vi "Unit 5M.vi"() -> ()   [LabVIEW 2023]
panel:
  out "isTrue":bool=TRUE
  in  "Мащаб 1 сек:1":u32=1000
  in  "k Минути":dbl format="%#_2g"
  out "Nк %":dbl format="%#_4g"
  out "Минути":dbl format="%#_2g"
  out "Час":i64
  out "tmp":dbl
  out "Часа":dbl format="%#_2g"
  out "Минути":dbl format="%#_4g"
  out "dN %/мин":dbl format="%#_2g"
  in  "dN/dT %/ h":dbl format="%#_2g"
  in  "N1 %":dbl format="%#_3g"
  out "Waveform Chart":T1(graph)
  out "N след 1 минута":dbl format="%#_4g"
  out "N текуща %":dbl format="%#_4g"
  in  "N2 %":dbl format="%#_3g"
  # "със"
  # "За"
  # "min"
  # "мил. сек."
  # "след"
  # "Общо време"
  # ":"
  # "="
  # "%"
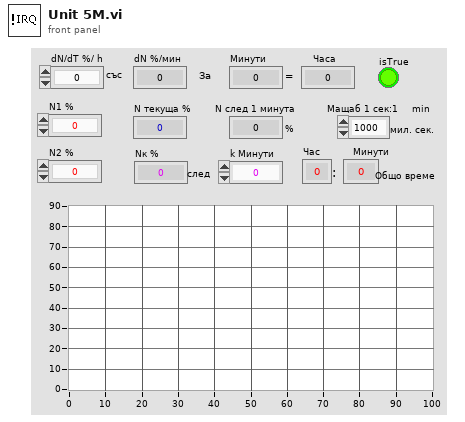
[diagram p1: front panel]
types:
  T1 = cluster{"N текуща % ":dbl, "N2 % ":dbl, "Nк %  ":dbl}
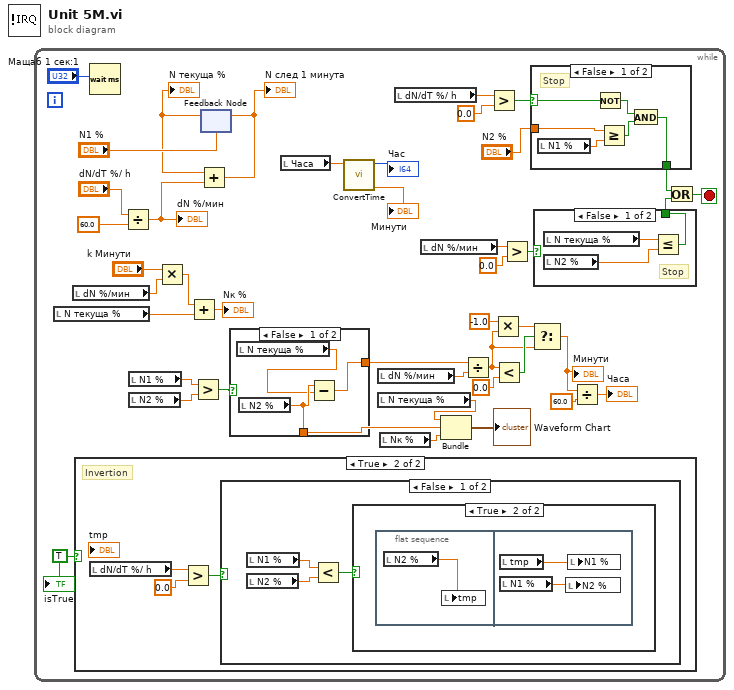
[diagram p0: block diagram]
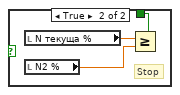
[diagram p2: hidden frame]
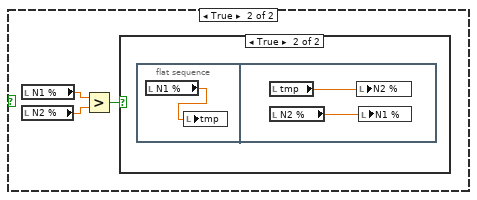
[diagram p5: hidden frame]
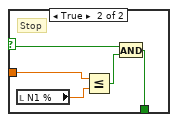
[diagram p7: hidden frame]
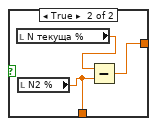
[diagram p8: hidden frame]
diagram:
  n1 = while {
    stop <- w6 stop-if-true
    w27 = TRUE
    n2 = local read "N текуща %"() -> (w9:dbl)
    n3 = local read "dN %/мин"() -> (w12:dbl)
    n4 = case shown="True" w27 {
      frame False {
      }
      frame True {
        # "Invertion"
        n5 = local read "dN/dT %/ h"() -> (w52:dbl)
        n6 = Greater?(x=w52, y=0.0) -> (0:w50:bool)
        n7 = case shown="False" w50 {
          frame False {
            n8 = local read "N1 %"() -> (w55:dbl)
            n9 = local read "N2 %"() -> (w54:dbl)
            n10 = Less?(x=w55, y=w54) -> (x < y?=w53:bool)
            n11 = case shown="True" w53 {
              frame False {
              }
              frame True {
                n12 = flat-sequence {
                  frame #0 {
                    n13 = local read "N2 %"() -> (w56:dbl)
                    n14 = local write "tmp"(w56) -> ()
                  }
                  frame #1 {
                    n15 = local read "tmp"() -> (w57:dbl)
                    n16 = local read "N1 %"() -> (w58:dbl)
                    n17 = local write "N2 %"(w58) -> ()
                    n18 = local write "N1 %"(w57) -> ()
                  }
                }
              }
            }
          }
          frame True {
            n19 = local read "N1 %"() -> (w61:dbl)
            n20 = local read "N2 %"() -> (w60:dbl)
            n21 = Greater?(x=w61, y=w60) -> (0:w59:bool)
            n22 = case shown="True" w59 {
              frame False {
              }
              frame True {
                n23 = flat-sequence {
                  frame #0 {
                    n24 = local read "N1 %"() -> (w62:dbl)
                    n25 = local write "tmp"(w62) -> ()
                  }
                  frame #1 {
                    n26 = local read "tmp"() -> (w64:dbl)
                    n27 = local read "N2 %"() -> (w63:dbl)
                    n28 = local write "N2 %"(w64) -> ()
                    n29 = local write "N1 %"(w63) -> ()
                  }
                }
              }
            }
          }
        }
      }
    }
    n30 = Wait (ms)(milliseconds to wait="Мащаб 1 сек:1") -> ()  [unwired: 1 out]
    n31 = Divide(x="dN/dT %/ h", y=60.0) -> (x/y=w40:dbl)
    "dN %/мин" <- w40
    n32 = local read "N1 %"() -> (w36:dbl)
    n33 = local read "N2 %"() -> (w35:dbl)
    n34 = Multiply(x="k Минути", y=w12) -> (x*y=w10:dbl)
    n35 = Add(x=w10, y=w9) -> (x+y=→"Nк %":dbl)
    n36 = Greater?(x=w36, y=w35) -> (0:w34:bool)
    n37 = feedback #1("N1 %") -> (w39:dbl)
    "N текуща %" <- w39
    n38 = Add(x=w39, y=w40) -> (x+y=w38:dbl)
    "N след 1 минута" <- w38
    n39 = feedback-in #1(w38) -> ()
    n40 = case shown="False" w34 {
      tunnel: [w78 w81] -> w33
      tunnel: [w77 w79] -> w30
      frame False {
        n41 = local read "N текуща %"() -> (w76:dbl)
        n42 = local read "N2 %"() -> (w77:dbl)
        n43 = Subtract(x=w77, y=w76) -> (x-y=w78:dbl)
      }
      frame True {
        n44 = local read "N текуща %"() -> (w80:dbl)
        n45 = local read "N2 %"() -> (w79:dbl)
        n46 = Subtract(x=w80, y=w79) -> (x-y=w81:dbl)
      }
    }
    n47 = local read "Часа"() -> (w26:dbl)
    n48 = call "ConvertTime.vi"("Час1"=w26) -> ("Минути"=→"Минути":dbl, "Час"=→"Час":i64)  [unwired: 9 in]
    n49 = local read "dN %/мин"() -> (w23:dbl)
    n50 = local read "N текуща %"() -> (w31:dbl)
    n51 = local read "Nк %"() -> (w1:dbl)
    n52 = local read "dN/dT %/ h"() -> (w14:dbl)
    n53 = local read "dN %/мин"() -> (w5:dbl)
    n54 = Bundle("N текуща %"=w31, "N2 %"=w30, "Nк %"=w1) -> (→"Waveform Chart":T1)  [unwired: 1 in]
    n55 = Divide(x=w33, y=w23) -> (x/y=w17:dbl)
    n56 = Greater?(x=w14, y=0.0) -> (0:w16:bool)
    n57 = Multiply(x=-1.0 ("y"), y=w17) -> (x*y=w20:dbl)
    n58 = Less?(x=w17, y=0.0) -> (x < y?=w21:bool)
    n59 = Greater?(x=w5, y=0.0) -> (0:w3:bool)
    n60 = case shown="False" w16 {
      selector: w16 -> [w66 w73]
      tunnel: [w68 w71] -> w8
      tunnel: "N2 %" -> [w67 w72]
      frame False {
        # "Stop"
        n61 = local read "N1 %"() -> (w69:dbl)
        n62 = Not(x=w66) -> (.not. x?=w65:bool)
        n63 = Greater Or Equal?(x=w67, y=w69) -> (x >= y?=w70:bool)
        n64 = And(x=w65, y=w70) -> (x .and. y?=w68:bool)
      }
      frame True {
        # "Stop"
        n65 = local read "N1 %"() -> (w74:dbl)
        n66 = Less Or Equal?(x=w72, y=w74) -> (x <= y?=w75:bool)
        n67 = And(x=w73, y=w75) -> (x .and. y?=w71:bool)
      }
    }
    n68 = Select(t=w20, s=w21, f=w17) -> (s? t:f=w19:dbl)
    "Минути" <- w19
    n69 = case shown="False" w3 {
      tunnel: [w46 w47] -> w7
      frame False {
        # "Stop"
        n70 = local read "N текуща %"() -> (w45:dbl)
        n71 = local read "N2 %"() -> (w44:dbl)
        n72 = Less Or Equal?(x=w45, y=w44) -> (x <= y?=w46:bool)
      }
      frame True {
        # "Stop"
        n73 = local read "N текуща %"() -> (w49:dbl)
        n74 = local read "N2 %"() -> (w48:dbl)
        n75 = Greater Or Equal?(x=w49, y=w48) -> (x >= y?=w47:bool)
      }
    }
    n76 = Divide(x=w19, y=60.0) -> (x/y=→"Часа":dbl)
    n77 = Or(x=w8, y=w7) -> (x .or. y?=w6:bool)
    "isTrue" <- w27
  }
